vi "Item_OnCommand.vi"(10 "Command ID":string, 11 "Object":T1) -> ()   [LabVIEW 2020, in "Actor Message Maker Provider.lvlib"]
uses:
  Actor Message Maker Provider.lvlib
  MessageMakerProvider/_Message Maker/Message Maker.lvlib
  MessageMakerProvider/_Message Maker/_Maker Classes/Abstract Message Scripter/Abstract Message Scripter.lvclass
  MessageMakerProvider/Support/Localized Strings.vi
  MessageMakerProvider/Message Maker Provider.lvlib
  <resource>/Framework/Providers/API/ItemRef.ctl
panel:
  out "error out":errorcluster
  in  "error in":errorcluster
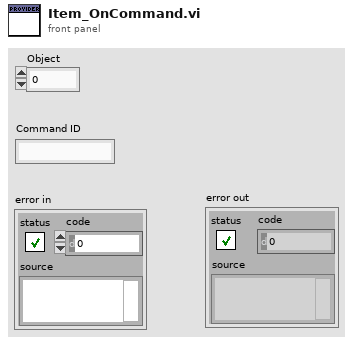
[diagram p1: front panel]
types:
  T1 = typedef "ItemRef.ctl" = u64
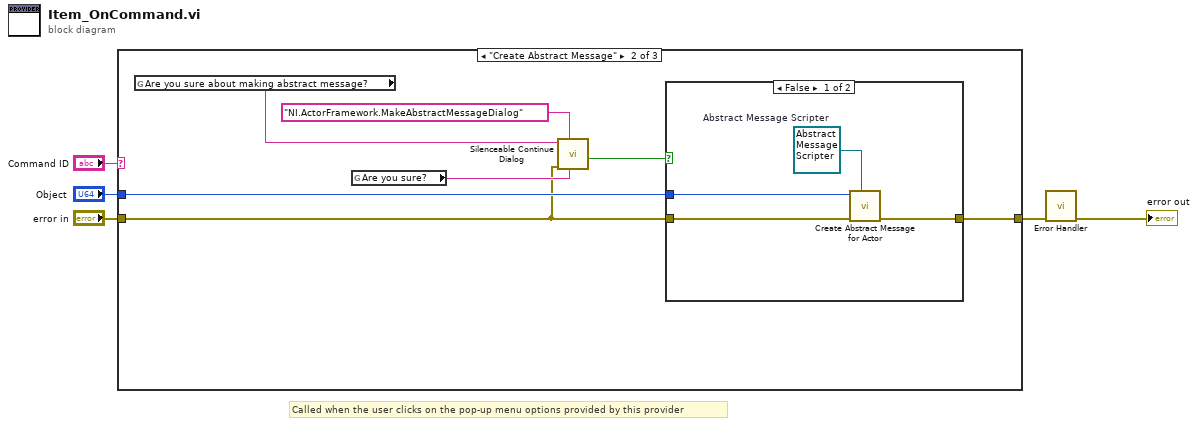
[diagram p0: block diagram]
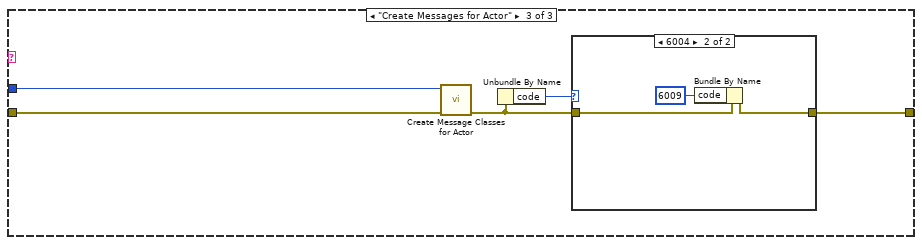
[diagram p4: hidden frame]
diagram:
  # "Called when the user clicks on the pop-up menu options provided by this provider"
  n1 = case shown="\"Create Abstract Message\"" "Command ID" {
    tunnel: "error in" -> [w6 w7 w23]
    tunnel: [w6 w13 w19] -> w2
    tunnel: "Object" -> [_ w12 w22]
    frame Default {
    }
    frame "Create Abstract Message" {
      n2 = global read "Localized Strings.vi" "Are you sure about making abstract message?"() -> (w11:string)
      n3 = global read "Localized Strings.vi" "Are you sure?"() -> (w8:string)
      n4 = call <vilib>:"Silenceable Continue Dialog.vi"("window title"=w8, "config key"="NI.ActorFramework.MakeAbstractMessageDialog", "error in (no error)"=w7, "message in"=w11) -> ("Cancelled?"=w9:bool)  [unwired: 6 in, 1 out]
      n5 = case shown="False" w9 {
        tunnel: w7 -> [w17 w18]
        tunnel: [w16 w18] -> w13
        tunnel: w12 -> [w15 _]
        frame False {
          w14 = refnum<class "Abstract Message Scripter.lvclass"> refnum  # Abstract Message Scripter
          n6 = call "Create Abstract Message for Actor.vi"("Abstract Message Scripter"=w14, "error in (no error)"=w17, "Object"=w15) -> ("error out"=w16:errorcluster)  [unwired: 8 in]
        }
        frame True {
        }
      }
    }
    frame "Create Messages for Actor" {
      n7 = call "Create Message Classes for Actor.vi"("error in (no error)"=w23, "Object"=w22) -> ("error out"=w20:errorcluster)  [unwired: 9 in]
      n8 = Unbundle By Name(w20) -> ("code"=w21:i32)
      n9 = case shown="6004" w21 {
        tunnel: w20 -> [w24 w27]
        tunnel: [w24 w26] -> w19
        frame 0, Default {
        }
        frame 6004 {
          n10 = Bundle By Name(cluster=w27, "code"=6009) -> (w26:errorcluster)
        }
      }
    }
  }
  n11 = call "Error Handler.vi"("error in (no error)"=w2) -> ("error out"=→"error out":errorcluster)  [unwired: 10 in]
